vi "Tachometer.vi"(11 "Enum":enum16{"Start", "Run", "End"}(ring)) -> (3 "RPM Current":dbl)   [LabVIEW 2012]
uses:
  TypeDefs/Digital Module 1.ctl
  <vilib>/Rock Robotics/SystemInterfaces/Typedef/FPGA_TypedefDigitalModule.ctl
  <vilib>/Rock Robotics/SystemInterfaces/DIO/FPGA_DIOChannel.ctl
  <vilib>/Rock Robotics/WPI/Counter/WPI_CounterDigitalInputToDigitalSource.vi
  <vilib>/Rock Robotics/WPI/Counter/WPI_CounterOpen Gear Tooth Sensor Mode.vi
  <vilib>/addons/control/pid/pid.llb/PID Control Input Filter (DBL).vi
  <vilib>/addons/control/pid/NI_PID_pid.lvlib
panel:
  out "Value":i32
  in  "MaxPeriod (sec)":dbl=0.1
  out "RPM Read":dbl(graph)
  in  "Digital Module A":T1={"Module"=enum."Digital Module 1", "Base Limit Switch"=enum."DIO 1", "Top Limit Switch"=enum."DIO 2", "Dummy Limit Switch"=enum."DIO 3", "Compressor Switch"=enum."DIO 4", "Tachometer"=enum."DIO 5", "Encoder A"=enum."DIO 6", "Encoder B"=enum."DIO 7", "Unassigned"=enum."DIO 8", "Unassigned"=enum."DIO 9", "Unassigned"=enum."DIO 10", "Unassigned"=enum."DIO 11", "Unassigned"=enum."DIO 12", "Unassigned"=enum."DIO 13", "Unassigned"=enum."DIO 14"}
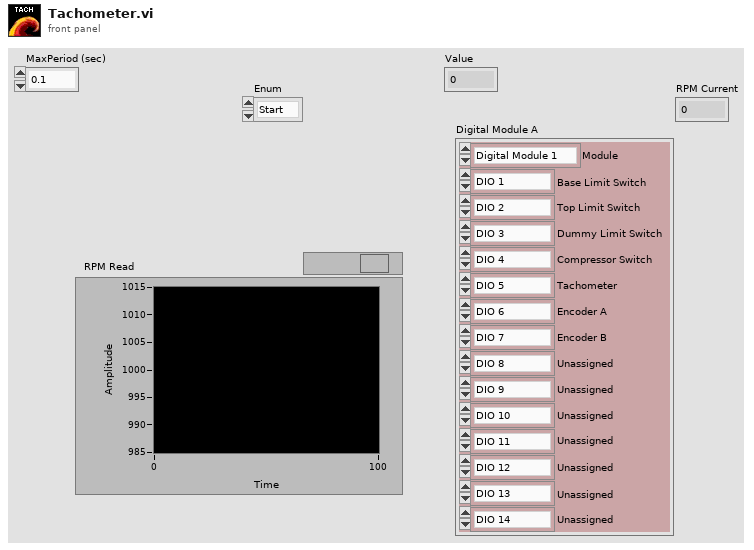
[diagram p1: front panel]
types:
  T1 = typedef "Digital Module 1.ctl" = cluster{"Module":T2, "Base Limit Switch":T3, "Top Limit Switch":T3, "Dummy Limit Switch":T3, "Compressor Switch":T3, "Tachometer":T3, "Encoder A":T3, "Encoder B":T3, "Unassigned":T3, "Unassigned":T3, "Unassigned":T3, "Unassigned":T3, "Unassigned":T3, "Unassigned":T3, "Unassigned":T3}
  T2 = typedef "FPGA_TypedefDigitalModule.ctl" = enum16{"Digital Module 1", "Digital Module 2"}
  T3 = typedef "FPGA_DIOChannel.ctl" = enum8{"DIO 1", "DIO 2", "DIO 3", "DIO 4", "DIO 5", "DIO 6", "DIO 7", "DIO 8", "DIO 9", "DIO 10", "DIO 11", "DIO 12", "DIO 13", "DIO 14", "Invalid"}
  T4 = typedef "WPI_DigitalInputDevRef.ctl" = cluster{"DevStatus":errorcluster, "DIO Channel":T3, "Digital Module":T2}
  T5 = typedef "FPGA_CounterEncoderSourceConvertionLVSourceType.ctl" = cluster{"DevStatus":errorcluster, "AnalogTriggerMode?":bool, "DigitalMode":cluster{"Digital Module":T2, "DIO Channel":T6}, "AnalogTriggerMode":cluster{"AnalogTriggerIndex":T7, "OutputType":T8}}
  T6 = typedef "FPGA_DIODigitalSourceChannel.ctl" = enum8{"DIO 1", "DIO 2", "DIO 3", "DIO 4", "DIO 5", "DIO 6", "DIO 7", "DIO 8", "DIO 9", "DIO 10", "DIO 11", "DIO 12", "DIO 13", "DIO 14", "Disabled"}
  T7 = typedef "FPGA_AnalogTriggerIndex.ctl" = enum8{"Trig 0", "Trig 1", "Trig 2", "Trig 3", "Trig 4", "Trig 5", "Trig 6", "Trig 7", "Invalid"}
  T8 = typedef "FPGA_AnalogTriggerOutType.ctl" = enum16{"InWindow", "TriggerState", "Rising", "Falling"}
  T9 = typedef "WPI_CounterDevRef.ctl" = cluster{"DevStatus":errorcluster, "CntIndex":T10}
  T10 = typedef "FPGA_CounterCtrSystemIndex.ctl" = enum8{"Ctr 0", "Ctr 1", "Ctr 2", "Ctr 3", "Ctr 4", "Ctr 5", "Ctr 6", "Ctr 7", "Invalid"}
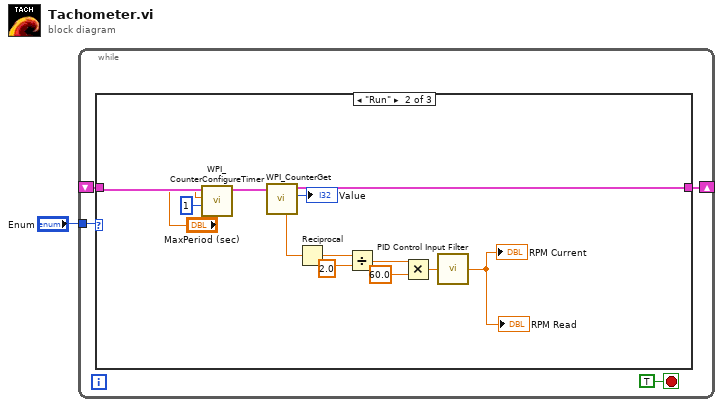
[diagram p0: block diagram]
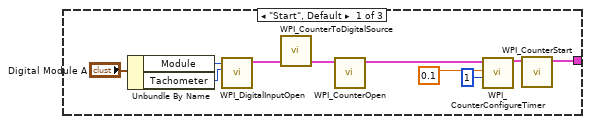
[diagram p2: hidden frame]
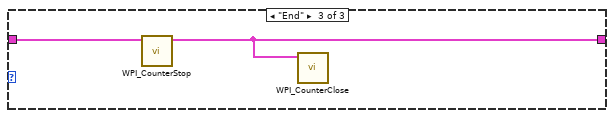
[diagram p3: hidden frame]
diagram:
  n1 = while {
    shift-right: [w5] -> _
    shift-left: _ -> [w4]
    tunnel: "Enum" -> [w2]
    stop <- TRUE stop-if-true
    n2 = case shown="\"Run\"" w2 {
      tunnel: [w12 w28 w29] -> w5
      tunnel: w4 -> [_ w20 w30]
      frame "Start", Default {
        n3 = Unbundle By Name("Digital Module A") -> ("Module"=w14:T2, "Tachometer"=w13:T3)
        n4 = call <vilib>:"WPI_DigitalInputOpen.vi"("DIO Channel"=w13, "Digital Module (Module 1)"=w14) -> ("DigitalInputDevRef"=w10:T4)  [unwired: 8 in, 1 out]
        n5 = call-poly <vilib>:"WPI_CounterToDigitalSource.vi"("DigitalInputDevRef"=w10) -> ("Digital Source"=w11:T5)  [unwired: 6 in]
        n6 = call-poly <vilib>:"WPI_CounterOpen.vi"("Source"=w11) -> ("CounterDevRef"=w9:T9)  [unwired: 9 in, 1 out]
        n7 = call <vilib>:"WPI_CounterConfigureTimer.vi"("Number Samples to Average"=u8 1, "MaxPeriod (sec)"=0.1, "CounterDevRef in"=w9) -> ("CounterDevRef out"=w8:T9)  [unwired: 7 in, 1 out]
        n8 = call <vilib>:"WPI_CounterStart.vi"("CounterDevRef in"=w8) -> ("CounterDevRef out"=w12:T9)  [unwired: 9 in, 1 out]
      }
      frame "Run" {
        n9 = call <vilib>:"WPI_CounterConfigureTimer.vi"("Number Samples to Average"=u8 1, "MaxPeriod (sec)"="MaxPeriod (sec)", "CounterDevRef in"=w20) -> ("CounterDevRef out"=w19:T9)  [unwired: 7 in, 1 out]
        n10 = call <vilib>:"WPI_CounterGet.vi"("CounterDevRef in"=w19) -> ("Value"=→"Value":i32, "CounterDevRef out"=w28:T9, "Period (sec)"=w24:dbl)  [unwired: 5 in, 3 out]
        n11 = Reciprocal(x=w24) -> (1/x=w23:dbl)
        n12 = Divide(x=w23, y=2.0) -> (x/y=w26:dbl)
        n13 = Multiply(x=w26, y=60.0) -> (x*y=w22:dbl)
        n14 = call-poly <vilib>:"PID Control Input Filter.vi"("input"=w22) -> ("output"=→"RPM Read" →"RPM Current":dbl)  [unwired: 4 in]
      }
      frame "End" {
        n15 = call <vilib>:"WPI_CounterStop.vi"("CounterDevRef in"=w30) -> ("CounterDevRef out"=w29:T9)  [unwired: 9 in, 1 out]
        n16 = call <vilib>:"WPI_CounterClose.vi"("CounterDevRef"=w29) -> ()  [unwired: 10 in, 1 out]
      }
    }
  }
